vi "Initialize SLSC Switch Engine.vi"(8 "error in (no error)":errorcluster, 11 "Device Ref in":T2 format="%.0x") -> (0 "error out":errorcluster, 1 "SLSC Switch Consumer out":refnum<class "SLSC Switch Consumer.lvclass">, 2 "FIFO Indices":T1, 3 "Device Ref out":T2 format="%.0x")   [LabVIEW 2017, in "SLSC Switch Engine.lvlib"]
uses:
  SLSC Switch Engine.lvlib
  <vilib>/NI Veristand/Custom Device API/Custom Device Item Ref.ctl
  Includes/SLSCSwitchMessaging.lvlibp/SLSC Switch Consumer/SLSC Switch Consumer.lvclass
  Shared/FIFO Indices.ctl
  Shared/Compiled.Settings.ctl
  Shared/Communication Configuration.ctl
  Shared/Driver Configuration.ctl
  Shared/Endpoint Configuration Cluster.ctl
  Shared/Endpoint Configuration Enum.ctl
  Includes/SLSCSwitchMessaging.lvlibp/SLSC Switch Init Parameters/SLSC Switch Init Parameters.lvclass
  C:/github/niveristand-routing-and-faulting-custom-device/Includes/CDMessaging.lvlibp/Parameters/Abstract Init Parameters/Abstract Init Parameters.lvclass
  C:/github/niveristand-routing-and-faulting-custom-device/Includes/CDMessaging.lvlibp/Switch/Abstract Switch Init Parameters/Abstract Switch Init Parameters.lvclass
  Includes/CDMessaging.lvlibp/Message Queue/Abstract Message Queue/Abstract Message Queue.lvclass
  Shared/Constants.vi
  <vilib>/NI Veristand/Custom Device API/Get Item Property (Variant).vi
  <vilib>/NI Veristand/Custom Device API/Custom Device API.lvlib
  Shared/SLSC Switch Shared.lvlib
  Includes/CDMessaging.lvlibp/Consumer/Abstract Consumer/Abstract Consumer.lvclass
  C:/github/niveristand-routing-and-faulting-custom-device/Includes/CDMessaging.lvlibp/Consumer/Abstract Consumer/Abstract Consumer.lvclass
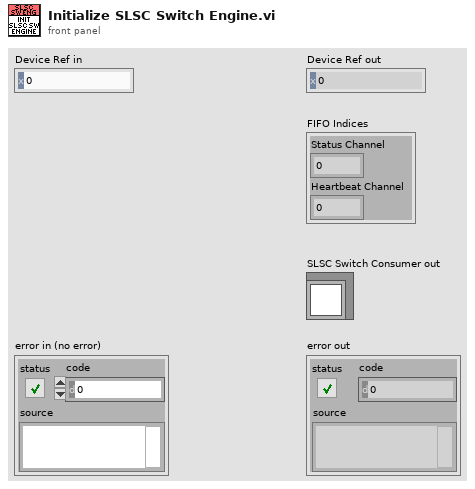
[diagram p1: front panel]
types:
  T1 = typedef "SLSC Switch Shared.lvlib/FIFO Indices.ctl" = cluster{"Status Channel":i32, "Heartbeat Channel":i32}
  T2 = typedef "Custom Device API.lvlib/Custom Device Item Ref.ctl" = u64
  T3 = typedef "SLSC Switch Shared.lvlib/Compiled.Settings.ctl" = cluster{"Custom Device Name":string, "Communication Configuration":T4, "Driver Configuration":T5, "FIFO Indices":T1}
  T4 = typedef "SLSC Switch Shared.lvlib/Communication Configuration.ctl" = cluster{"Consumer Queue Name":string}
  T5 = typedef "SLSC Switch Shared.lvlib/Driver Configuration.ctl" = cluster{"Resource Name":string, "Topology":string, "Switches JSON":string, "Endpoint Configuration":T6[]}
  T6 = typedef "SLSC Switch Shared.lvlib/Endpoint Configuration Cluster.ctl" = cluster{"Endpoint":string, "Configuration":T7}
  T7 = typedef "SLSC Switch Shared.lvlib/Endpoint Configuration Enum.ctl" = enum16{"Load", "Source", "Configuration"}
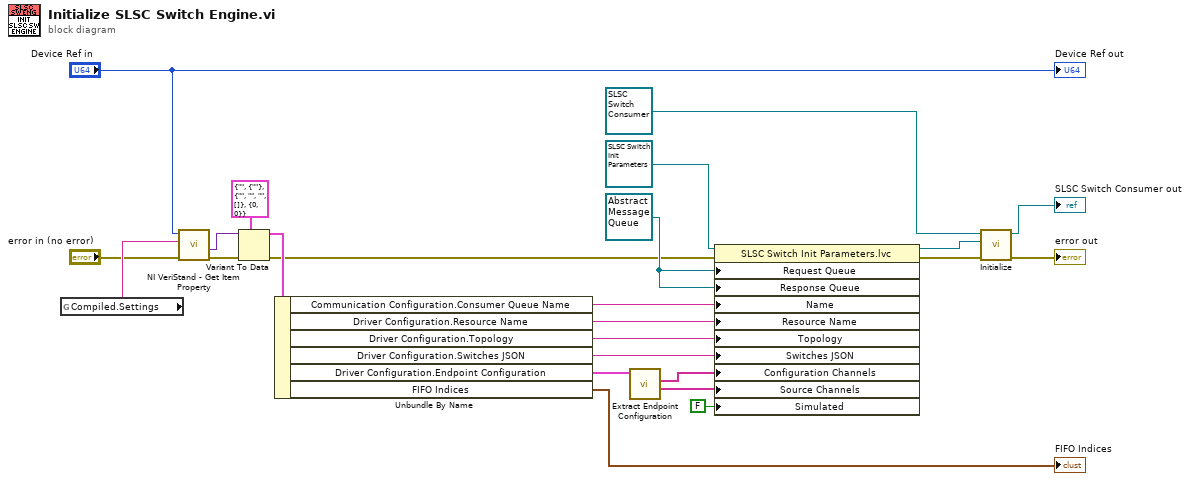
[diagram p0: block diagram]
diagram:
  w19 = refnum<class "Abstract Message Queue.lvclass"> refnum ("Request Queue")
  n1 = global read "Constants.vi" "Compiled.Settings"() -> (w24:string)
  n2 = call-poly <vilib>:"NI VeriStand - Get Item Property.vi"("error in (no error)"="error in (no error)", "Property Name"=w24, "Item Ref in"="Device Ref in") -> ("error out"=w23:errorcluster, "Value"=w22:variant)  [unwired: 5 in, 2 out]
  n3 = Variant To Data(error in=w23, type=T3 {"Custom Device Name"="", "Communication Configuration"={"Consumer Queue Name"=""}, "Driver Configuration"={"Resource Name"="", "Topology"="", "Switches JSON"="", "Endpoint Configuration"=[]}, "FIFO Indices"={"Status Channel"=0, "Heartbeat Channel"=0}} ("Compiled.Settings"), Variant=w22) -> (data=w17:T3, error out=w16:errorcluster)
  n4 = Unbundle By Name(w17) -> ("Communication Configuration.Consumer Queue Name"=w15:string, "Driver Configuration.Resource Name"=w14:string, "Driver Configuration.Topology"=w13:string, "Driver Configuration.Switches JSON"=w12:string, "Driver Configuration.Endpoint Configuration"=w3:T6[], "FIFO Indices"=→"FIFO Indices":T1)
  n5 = call "Extract Endpoint Configuration.vi"("Endpoint Configuration"=w3) -> ("Source Channels"=w1:string[], "Configuration Channels"=w2:string[])  [unwired: 8 in, 1 out]
  n6 = property class="SLSC Switch Init Parameters.lvc"(reference=refnum<class "SLSC Switch Init Parameters.lvclass"> refnum ("SLSC Switch Init Parameters"), error in=w16, "Request Queue"=w19, "Response Queue"=w19, "Name"=w15, "Resource Name"=w14, "Topology"=w13, "Switches JSON"=w12, "Configuration Channels"=w2, "Source Channels"=w1, "Simulated"=FALSE) -> (reference out=w8:refnum<class "SLSC Switch Init Parameters.lvclass">, error out=w10:errorcluster)
  n7 = call "Initialize.vi"("error in (no error)"=w10, "Parameters in"=w8, "Abstract Consumer in"=refnum<class "SLSC Switch Consumer.lvclass"> refnum ("SLSC Switch Consumer")) -> ("error out"=→"error out":errorcluster, "Abstract Consumer out"=→"SLSC Switch Consumer out":refnum<class "SLSC Switch Consumer.lvclass">)  [unwired: 7 in]
  "Device Ref out" <- "Device Ref in"
